vi "SDSU_ExposureLoop.vi"(5 "idle time":u32, 6 "stop ref":refnum<vi>, 7 "Total image bytes":u32, 8 "error IO":errorcluster, 9 "fast":bool, 10 "Database RefNum in":T1, 11 "SDSU_fd":i32) -> (0 "error out":errorcluster)   [LabVIEW 2016]
uses:
  DBSHAND/private/vis/DatabaseHand_RefNum.ctl
  Common/public/vis/CMN_FVAR_action.ctl
  DBSHAND/private/vis/DatabaseHand_Element_Get(I32).vi
  DBSHAND/private/vis/DatabaseHand_Element_Set(bool).vi
  c/lib/libarcDHE.so
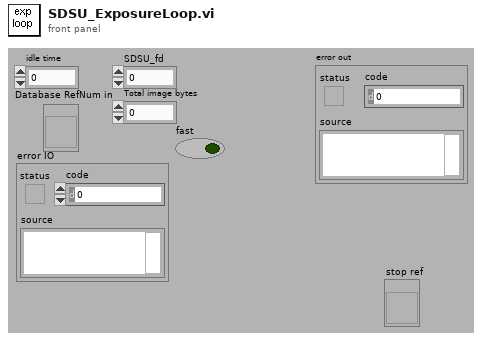
[diagram p1: front panel]
types:
  T1 = typedef "DatabaseHand_RefNum.ctl" = refnum<vi>
  T2 = typedef "CMN_ContStatus.ctl" = cluster{"Response":string, "power":bool, "shutter":bool, "artifdata":bool, "idlemode":bool, "reset":bool, "gain":u8, "speed":u8, "resetPCI":bool, "autoshutter":bool, "TempSetPoint":i32, "multipleextensions":bool, "displayImage":bool, "coadding":bool, "images being coadded":i32, "Operation Mode":enum16{"normal", "coadd", "fawler"}, "frames to write":cluster{"subs":bool, "reset":bool, "exposed":bool}, "fawler samples":i32, "write auto":bool, "datatype":string, "frames to display":cluster{"subs":bool, "reset":bool, "exposed":bool}, "sur":i32, "autoclear":bool}
  T3 = typedef "CMN_FVAR_action.ctl" = enum16{"read", "write"}
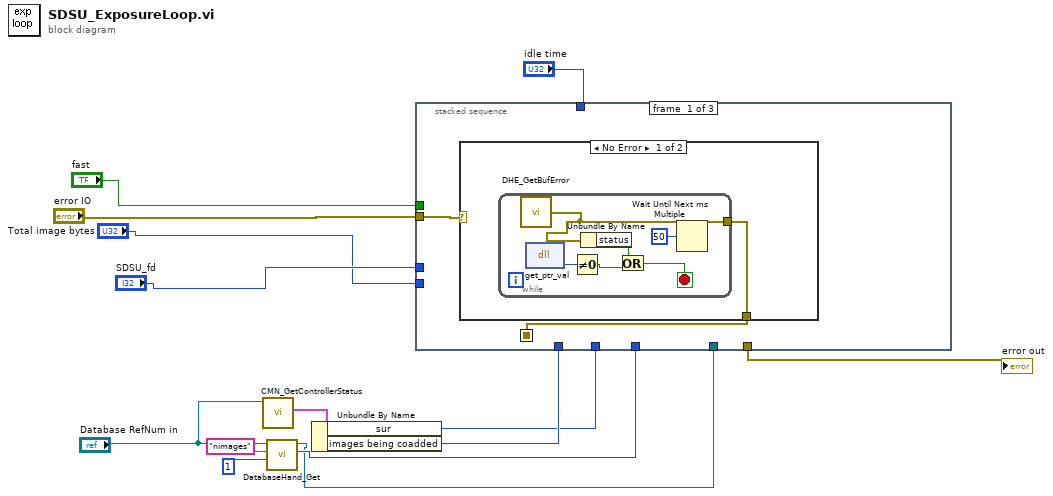
[diagram p0: block diagram]
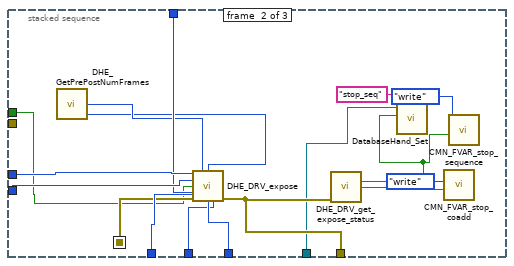
[diagram p3: hidden frame]
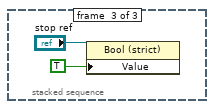
[diagram p4: hidden frame]
diagram:
  n1 = call "CMN_GetControllerStatus.vi"("DBS Ref"="Database RefNum in") -> ("ControllerStatus"=w12:T2)  [unwired: 10 out]
  n2 = call-poly "DatabaseHand_Get.vi"("default value"=1, "name"="nimages", "Database RefNum in"="Database RefNum in") -> ("value"=w8:i32, "Database RefNum out"=w2:T1)  [unwired: 2 in, 5 out]
  n3 = Unbundle By Name(w12) -> ("sur"=w11:i32, "images being coadded"=w14:i32)
  n4 = stacked-sequence {
    seq-local: [w16 _ _] -> [_ w37 _]
    tunnel: "Total image bytes" -> [_ w40 _]
    tunnel: "SDSU_fd" -> [_ w41 _]
    tunnel: [_ w35 _] -> w13
    tunnel: "error IO" -> [w15 _ _]
    tunnel: w8 -> [_ w39 _]
    tunnel: w14 -> [_ w38 _]
    tunnel: "idle time" -> [_ w36 _]
    tunnel: w11 -> [_ w34 _]
    tunnel: "fast" -> [_ w26 _]
    tunnel: w2 -> [_ w25 _]
    frame #0 {
      n5 = case shown="No Error" w15 {
        selector: w15 -> [_ w24]
        tunnel: [w17 w24] -> w16
        frame No Error {
          n6 = while {
            tunnel: [w18] -> w17
            stop <- w20 stop-if-true
            n7 = call "DHE_GetBufError.vi"() -> ("DHE_BufError"=w18:errorcluster)  [unwired: 9 out]
            n8 = dll-call lib="home/simager/panview/PAN/Modules/SDSU/private/c/lib/libarcDHE.so" fn="get_ptr_val"() -> ("return type"=w23:u64)  [unwired: 3 in, 2 out]
            n9 = Not Equal To 0?(x=w23) -> (x != 0?=w22:bool)
            n10 = Unbundle By Name(w18) -> ("status"=w19:bool)
            n11 = Or(x=w19, y=w22) -> (x .or. y?=w20:bool)
            n12 = Wait Until Next ms Multiple(millisecond multiple=u32 50) -> ()  [unwired: 1 out]
          }
        }
        frame Error {
        }
      }
    }
    frame #1 {
      n13 = call "DHE_GetPrePostNumFrames.vi"() -> ("DHE_PreExpose"=w32:i32, "DHE_PostExpose"=w31:i32)  [unwired: 8 out]
      n14 = call "DHE_DRV_expose.vi"("fd"=w41, "num_prevex"=w32, "num_postex"=w31, "bytes_to_receive"=w40, "fast"=w26, "expt_time"=w36, "error in (no error)"=w37, "num_coadds"=w38, "npics"=w39, "num_sur"=w34) -> ("error out"=w35:errorcluster)  [unwired: 5 out]
      n15 = call "DHE_DRV_get_expose_status.vi"("error in (no error)"=w35) -> ("sequence stoped"=w30:bool, "coadd stoped"=w28:bool)  [unwired: 13 out]
      n16 = call-poly "DatabaseHand_Set.vi"("name"="stop_seq", "value"=w30, "Database RefNum in"=w25) -> ()  [unwired: 5 in, 4 out]
      n17 = call "CMN_FVAR_stop_coadd.vi"("value in"=w28, "action"=CMN_FVAR_action."write") -> ()  [unwired: 9 out]
      n18 = call "CMN_FVAR_stop_sequence.vi"("value in"=w30, "action"=CMN_FVAR_action."write") -> ()  [unwired: 9 out]
    }
    frame #2 {
      n19 = property class="Bool (strict)"(reference="stop ref", "Value"=TRUE) -> ()  [unwired: 1 in, 2 out]
    }
  }
  "error out" <- w13
